vi "SR430_initialize.vi"(0 "SR430 VISA Cluster":T1, 5 "Revision Query (F: Check)":bool, 11 "error in (no error)":errorcluster) -> (4 "SR430 VISA Cluster out":T1, 6 "Revision":string, 8 "interface initialized":bool, 15 "error out":errorcluster)   [LabVIEW 2015, in "SR430Driver.lvlib"]
doc: "This VI passes the addressing information in the instrument decriptor to the Instr Open VI and returns the instrument ID. You must run this VI before using any of the instrument driver VIs for this instrument.\n\nCopyright (C) \nGesellschaft f. Schwerionenforschung, GSI\nPlanckstr. 1\n64291 Darmstadt\nGermany\n\nContact: http://www-wnt.gsi.de/labview, d.beck@gsi.de\n\nThis program is free software; you can redistribute it and/or\nmodify it under the terms of the GNU General Public License\nas published by the Free Software Foundation; either version 2\nof the License, or (at your option) any later version.\n\nThis program is distributed in the hope that it will be useful,\nbut WITHOUT ANY WARRANTY; without even the implied warranty of\nMERCHANTABILITY or FITNESS FOR A PARTICULAR PURPOSE. See the\nGNU General Public License for more details (http://www.gnu.org)."
uses:
  SR430Driver.lvlib
  SR430_VISA Control.ctl
panel:
  # "Check\nDon't Check"
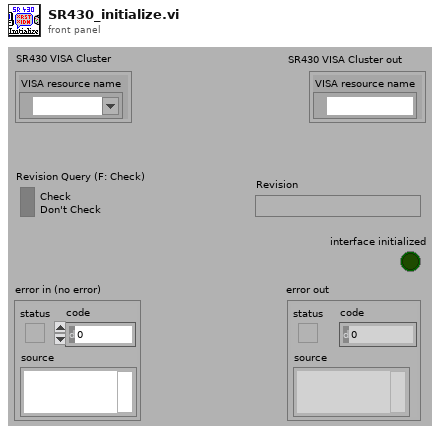
[diagram p1: front panel]
types:
  T1 = typedef "SR430Driver.lvlib/SR430_VISA Control.ctl" = cluster{"VISA resource name":refnum<visa-resource-name>}
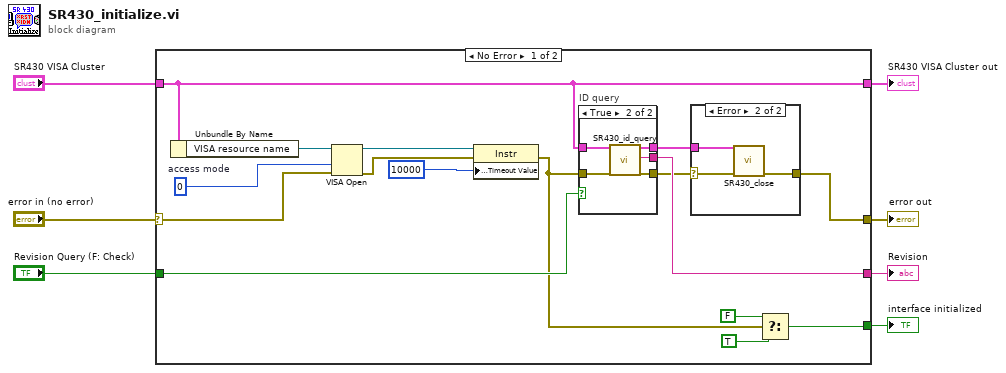
[diagram p0: block diagram]
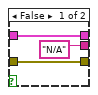
[diagram p3: hidden frame]
diagram:
  n1 = case shown="No Error" "error in (no error)" {
    selector: "error in (no error)" -> [w16 w36]
    tunnel: "Revision Query (F: Check)" -> [w23 _]
    tunnel: [w9 w36] -> w6
    tunnel: "SR430 VISA Cluster" -> [w12 w37]
    tunnel: [w12 w37] -> w4
    tunnel: [w20 _] -> w3
    tunnel: [w17 _] -> w2
    frame No Error {
      w22 = u32 0  # access mode
      n2 = Unbundle By Name(w12) -> ("VISA resource name"=w21:refnum<visa-resource-name>)
      n3 = VISA Open(access mode=w22, error in (no error)=w16, VISA resource name=w21) -> (VISA resource name=w15:refnum<visa-resource-name>, error out=w14:errorcluster)  [unwired: 2 in]
      n4 = property on="Property Node" class="Instr"(reference=w15, error in=w14, "General Settings:Timeout Value"=u32 10000) -> (error out=w8:errorcluster)  [unwired: 1 out]
      n5 = case "ID query" shown="True" w23 {
        tunnel: [w30 w33] -> w11
        tunnel: w8 -> [w30 w34]
        tunnel: w12 -> [w28 w35]
        tunnel: ["N/A" ("Revision") w32] -> w20
        tunnel: [w28 w31] -> w10
        frame False {
        }
        frame True {
          n6 = call "SR430_id_query.vi"("address"=w35, "error in (no error)"=w34) -> ("address out"=w31:T1, "identification string"=w32:string, "error out"=w33:errorcluster)  [unwired: 15 in]
        }
      }
      n7 = case shown="Error" w11 {
        selector: w11 -> [w24 w27]
        tunnel: w10 -> [_ w26]
        tunnel: [w24 w25] -> w9
        frame No Error {
        }
        frame Error {
          n8 = call "SR430_close.vi"("SR430 VISA Cluster"=w26, "error in (no error)"=w27) -> ("error out"=w25:errorcluster)  [unwired: 13 in]
        }
      }
      n9 = Select(t=FALSE, s=w8, f=TRUE) -> (s? t:f=w17:bool)
    }
    frame Error {
    }
  }
  "error out" <- w6
  "SR430 VISA Cluster out" <- w4
  "Revision" <- w3
  "interface initialized" <- w2
